vi "Get Slaves Number & Positions.vi"(8 "error in (no error)":errorcluster, 11 "VISA resource name":refnum<visa-resource-name>) -> (0 "error out":errorcluster, 1 "Connected Slaves":bool[](array[boolean]), 2 "No. of Slaves":u32, 3 "VISA resource name out":refnum<visa-resource-name>)   [LabVIEW 2020, in "QuPMXdriver.lvlib"]
doc: "Returns number of slaves connected to the master board, and positions of the slaves."
uses:
  QuPMXdriver.lvlib
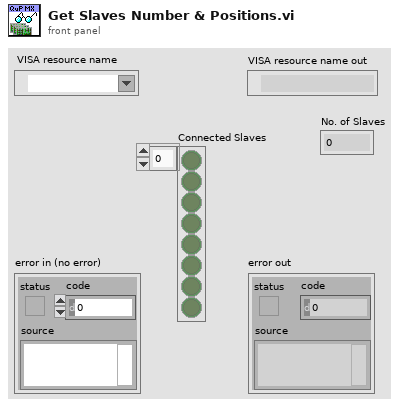
[diagram p1: front panel]
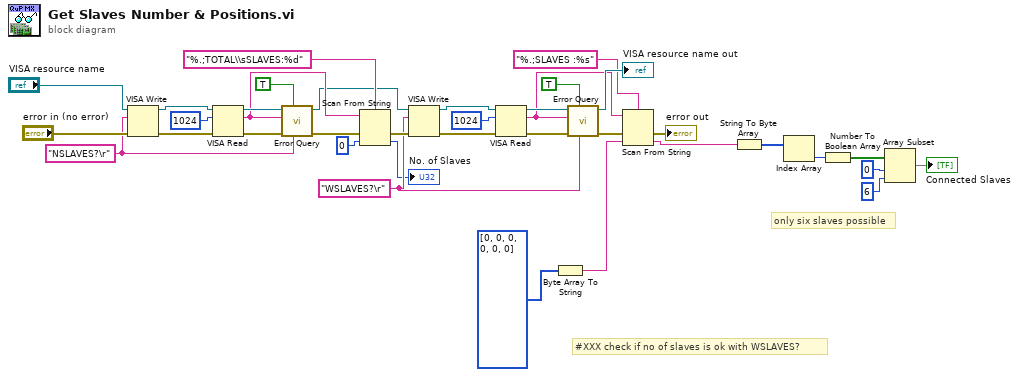
[diagram p0: block diagram]
diagram:
  w15 = "WSLAVES?\r"
  w27 = "NSLAVES?\r"
  # "only six slaves possible"
  # "#XXX check if no of slaves is ok with WSLAVES?"
  n1 = VISA Write(VISA resource name="VISA resource name", write buffer=w27, error in (no error)="error in (no error)") -> (VISA resource name out=w33:refnum<visa-resource-name>, error out=w26:errorcluster)  [unwired: 1 out]
  n2 = VISA Read(VISA resource name=w33, byte count=u32 1024, error in (no error)=w26) -> (VISA resource name out=w32:refnum<visa-resource-name>, read buffer=w28:string, error out=w31:errorcluster)  [unwired: 1 out]
  n3 = call "Error Query.vi"("Last command"=w27, "Ignore empty sequence? (T)"=TRUE, "error in (no error)"=w31, "Read buffer"=w28, "VISA resource name"=w32) -> ("error out"=w29:errorcluster, "VISA resource name out"=w18:refnum<visa-resource-name>)  [unwired: 5 in]
  n4 = Scan From String(format string="%.;TOTAL\\sSLAVES:%d", input string=w28, error in=w29, default 1=u32 0 ("default value 1")) -> (error out=w17:errorcluster, output 1=→"No. of Slaves":u32)  [unwired: 1 in, 2 out]
  n5 = VISA Write(VISA resource name=w18, write buffer=w15, error in (no error)=w17) -> (VISA resource name out=w20:refnum<visa-resource-name>, error out=w24:errorcluster)  [unwired: 1 out]
  n6 = VISA Read(VISA resource name=w20, byte count=u32 1024, error in (no error)=w24) -> (VISA resource name out=w21:refnum<visa-resource-name>, read buffer=w11:string, error out=w22:errorcluster)  [unwired: 1 out]
  n7 = Byte Array To String(unsigned byte array=u8[] [0, 0, 0, 0, 0, 0]) -> (string=w6:string)
  n8 = call "Error Query.vi"("Last command"=w15, "Ignore empty sequence? (T)"=TRUE, "error in (no error)"=w22, "Read buffer"=w11, "VISA resource name"=w21) -> ("error out"=w9:errorcluster, "VISA resource name out"=→"VISA resource name out":refnum<visa-resource-name>)  [unwired: 5 in]
  n9 = Scan From String(format string="%.;SLAVES :%s", input string=w11, error in=w9, default 1=w6) -> (error out=→"error out":errorcluster, output 1=w5:string)  [unwired: 1 in, 2 out]
  n10 = String To Byte Array(string=w5) -> (unsigned byte array=w13:u8[])
  n11 = Index Array(array=w13) -> (element=w12:u8)  [unwired: 1 in]
  n12 = Number To Boolean Array(number=w12) -> (Boolean array=w4:bool[])
  n13 = Array Subset(array=w4, index=0, length=6) -> (→"Connected Slaves":bool[])
